vi "IV_curve_plot.vi"(2 "I":dbl[](array[numeric]), 3 "V":dbl[](array[numeric])) -> (9 "Resistance":dbl, 10 "Offset":dbl)   [LabVIEW 2014]
uses:
  <vilib>/Analysis/NI_AALPro.lvlib
panel:
  out "IV measurement":cluster{"I":dbl[], "V":dbl[]}(graph)
  # "Raw Output"
  # "MOhms"
  # "mV"
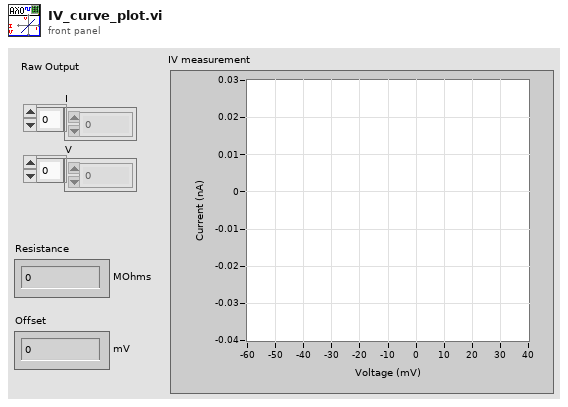
[diagram p1: front panel]
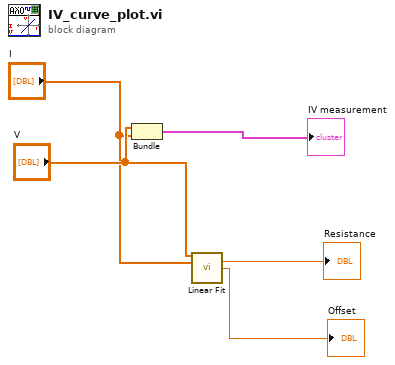
[diagram p0: block diagram]
diagram:
  n1 = Bundle("V"="V", "I"="I") -> (→"IV measurement":cluster{"V":dbl[], "I":dbl[]})  [unwired: 1 in]
  n2 = call <vilib>:"Linear Fit.vi"("Y"="V", "X"="I") -> ("slope"=→"Resistance":dbl, "intercept"=→"Offset":dbl)  [unwired: 9 in, 3 out]
